vi "TC1016_DEMO.vi"() -> ()   [LabVIEW 2019]
uses:
  SubVI/Typedef/TLibLIN.ctl
panel:
  out "Connect_TSLIN_Successfully":bool
  in  "退出程序":bool
  in  "打开LIN":bool
  in  "选项卡控件":T1(tab)
  in  "TLIBLIN 2":T2
  in  "LIN1_Write":bool
  in  "LIN1_ABaudrateKbps":sgl=19.2 format="%#_g  k"
  in  "LIN1_AProtocol":i32(ring)=2 items=["Lin_Protocol_13", "Lin_Protocol_20", "Lin_Protocol_21", "Lin_Protocol_J2602"]
  in  "LIN1_AHwChannel":i32(ring) items=["CHN1", "CHN2", "CHN3", "CHN4", "CHN5", "CHN6", "CHN7", "CHN8", "CHN9", "CHN10", "CHN11", "CHN12", "CHN13", "CHN14", "CHN15", "CHN16", "CHN17", "CHN18", "CHN19", "CHN20", "CHN21", "CHN22", "CHN23", "CHN24", "CHN25", "CHN26", "CHN27", "CHN28", "CHN29", "CHN30", "CHN31", "CHN32"]
  in  "LIN1_AAppChannel":i32(ring) items=["CHN1", "CHN2", "CHN3", "CHN4", "CHN5", "CHN6", "CHN7", "CHN8", "CHN9", "CHN10", "CHN11", "CHN12", "CHN13", "CHN14", "CHN15", "CHN16", "CHN17", "CHN18", "CHN19", "CHN20", "CHN21", "CHN22", "CHN23", "CHN24", "CHN25", "CHN26", "CHN27", "CHN28", "CHN29", "CHN30", "CHN31", "CHN32"]
  in  "LIN1_SetNode":i32(ring) items=["MasterNode", "SlaveNode", "MonitorNote"]
  in  "启用4通道":bool
  in  "启用3通道":bool
  in  "启用2通道":bool
  in  "启用1通道":bool
  in  "使用通道数量":u16(ring)=1 items=["1通道"=1, "2通道"=2, "3通道"=3, "4通道"=4, "5通道"=5]
  # "TC_1026_DEMO"
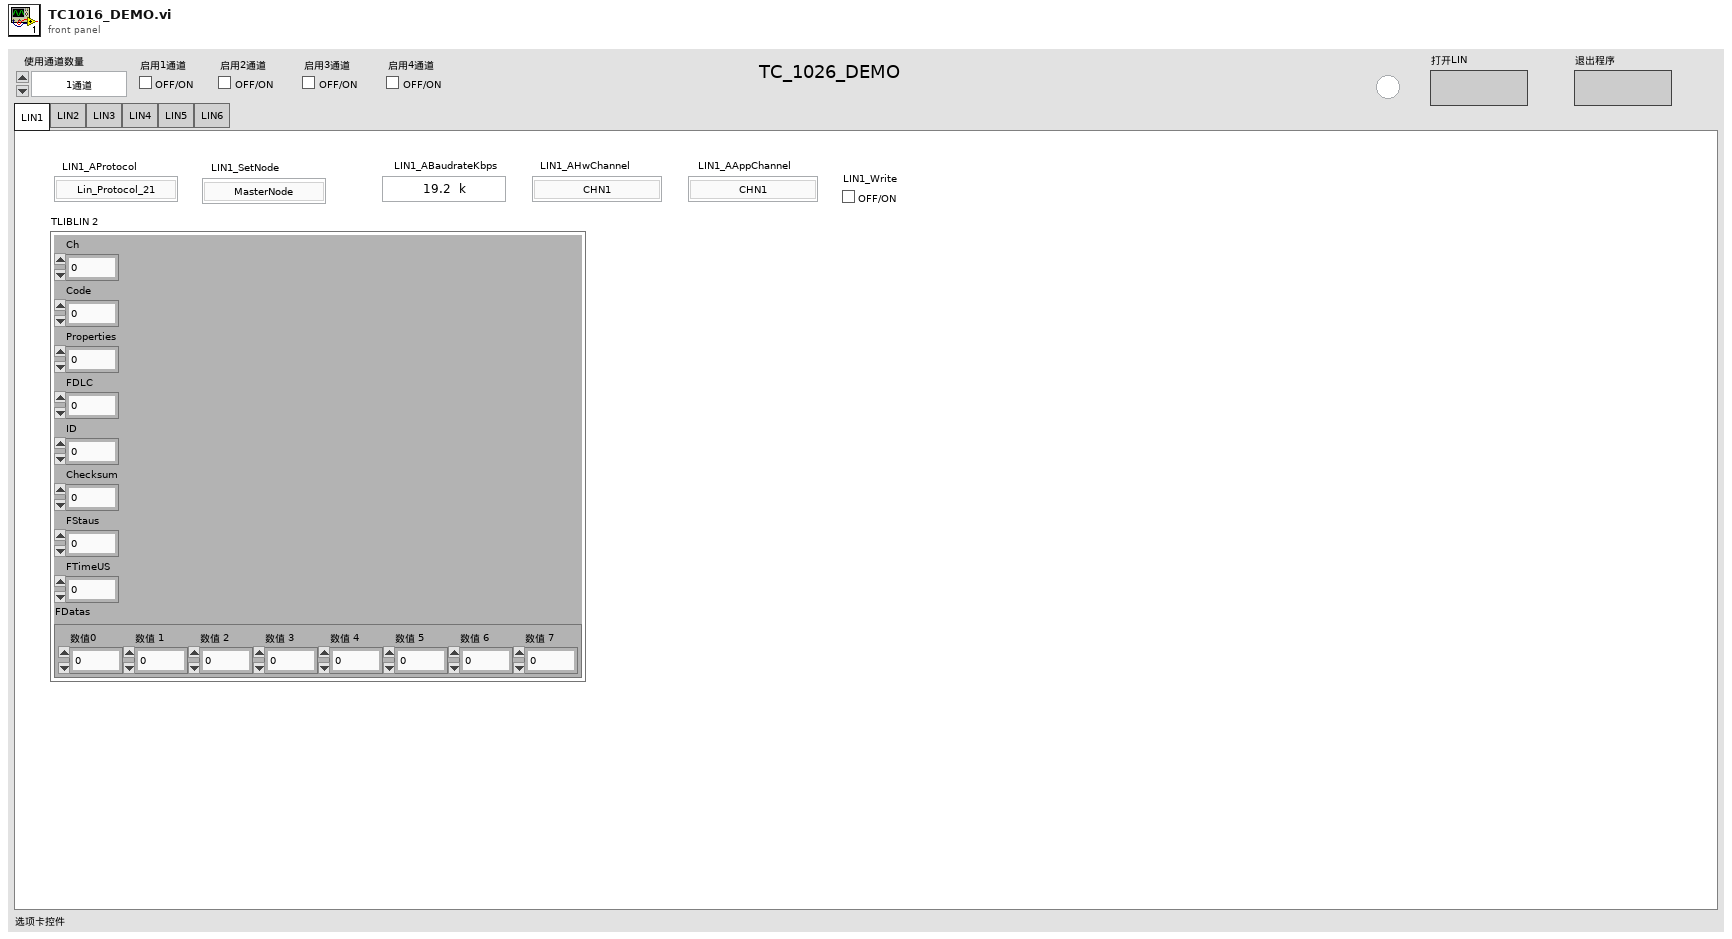
[diagram p1: front panel]
types:
  T1 = enum32{"LIN1", "LIN2", "LIN3", "LIN4", "LIN5", "LIN6"}
  T2 = typedef "TLibLIN.ctl" = cluster{"Ch":u8, "Code":u8, "Properties":u8, "FDLC":u8, "ID":u8, "Checksum":u8, "FStaus":u8, "FTimeUS":u64, "FDatas":cluster{"数值0":u8, "数值 1":u8, "数值 2":u8, "数值 3":u8, "数值 4":u8, "数值 5":u8, "数值 6":u8, "数值 7":u8}}
  T3 = cluster{"硬件类型":i32, "硬件子类型":i32, "AHwChannel":i32, "AAppChannel":i32, "ABaudrateKbps":sgl, "AProtocol":i32}
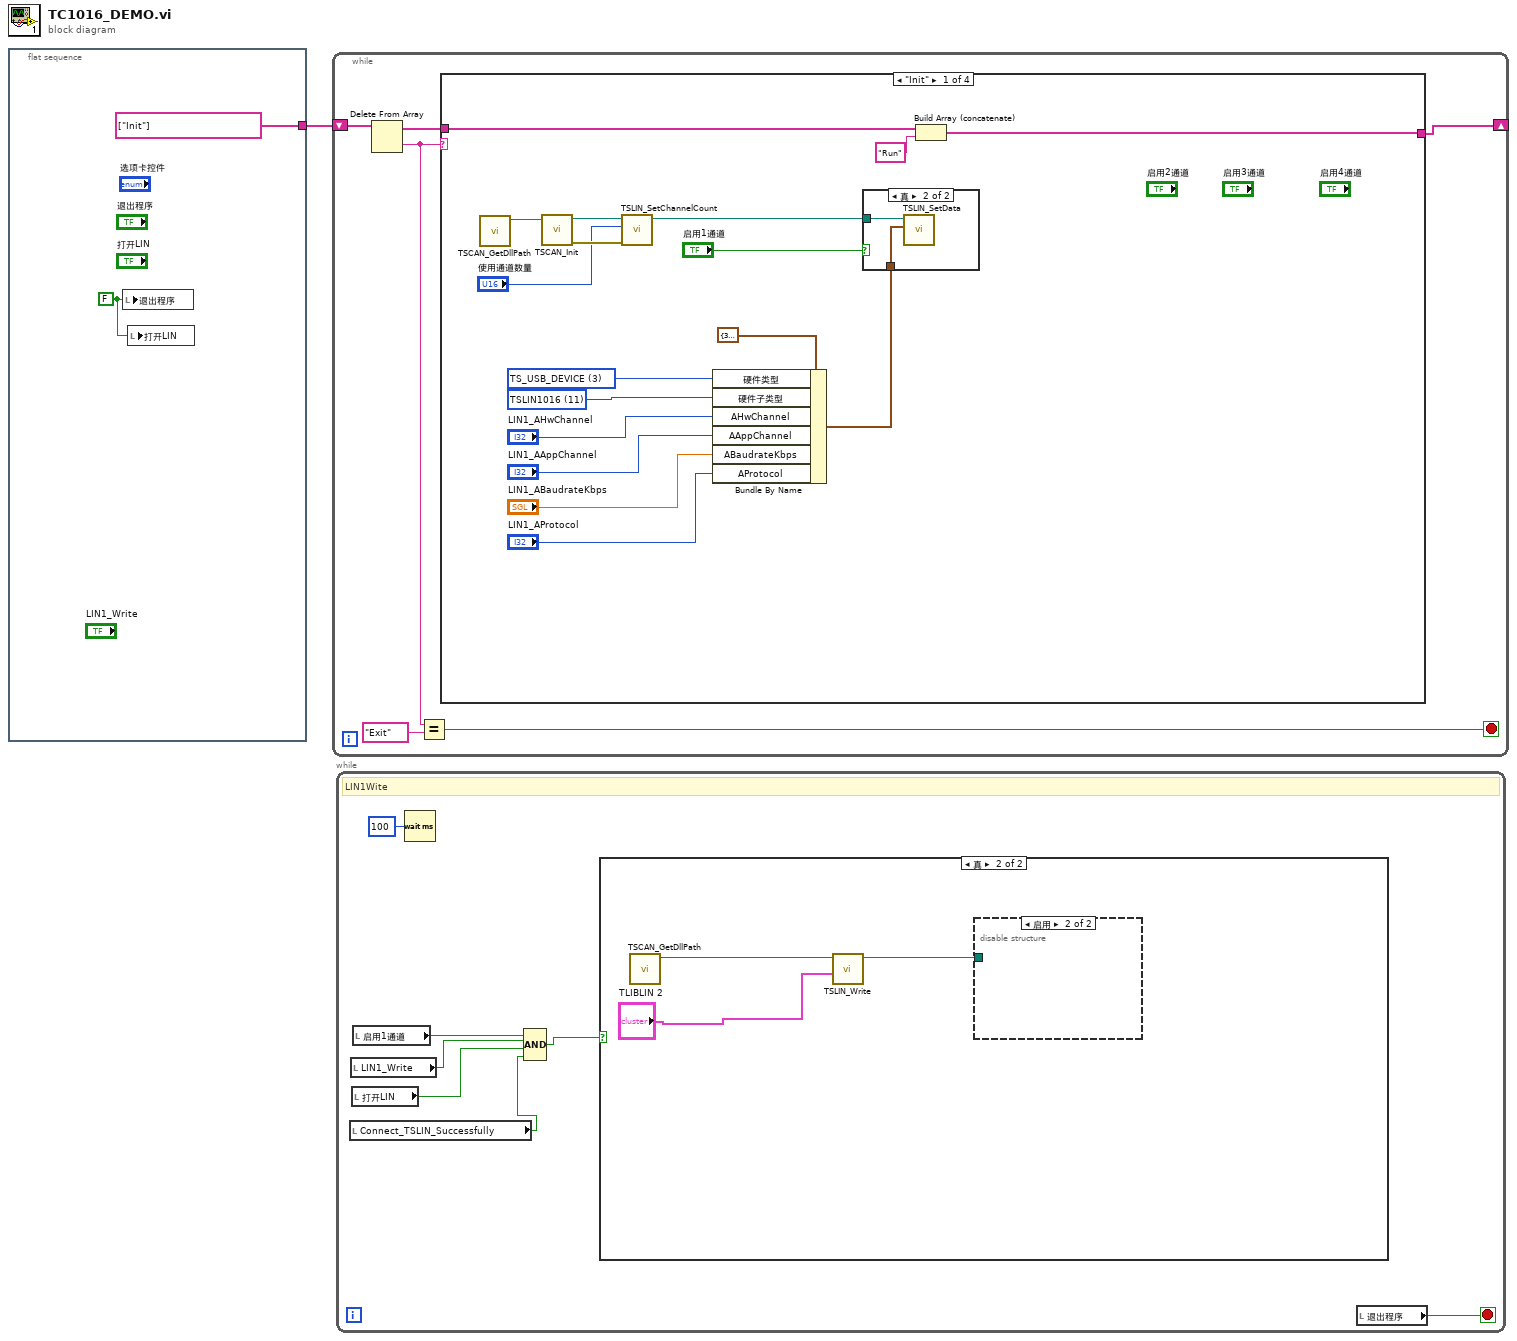
[diagram p0: block diagram]
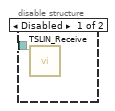
[diagram p3: hidden frame]
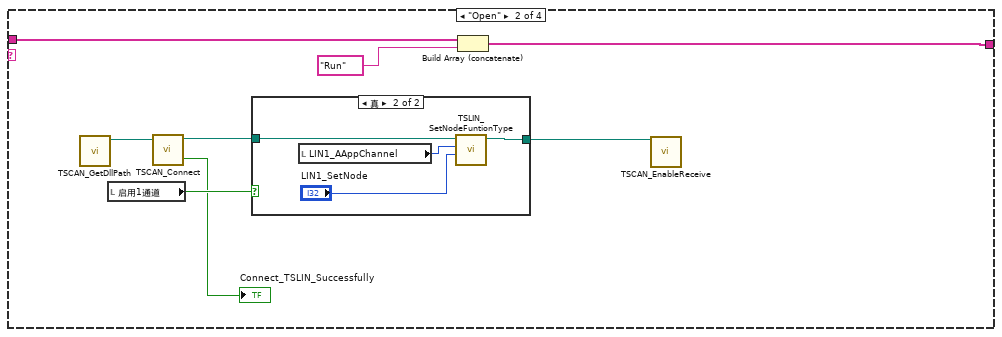
[diagram p5: hidden frame]
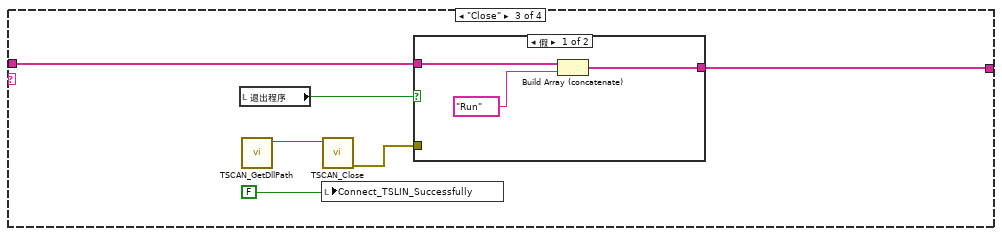
[diagram p7: hidden frame]
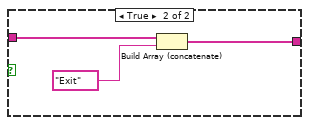
[diagram p8: hidden frame]
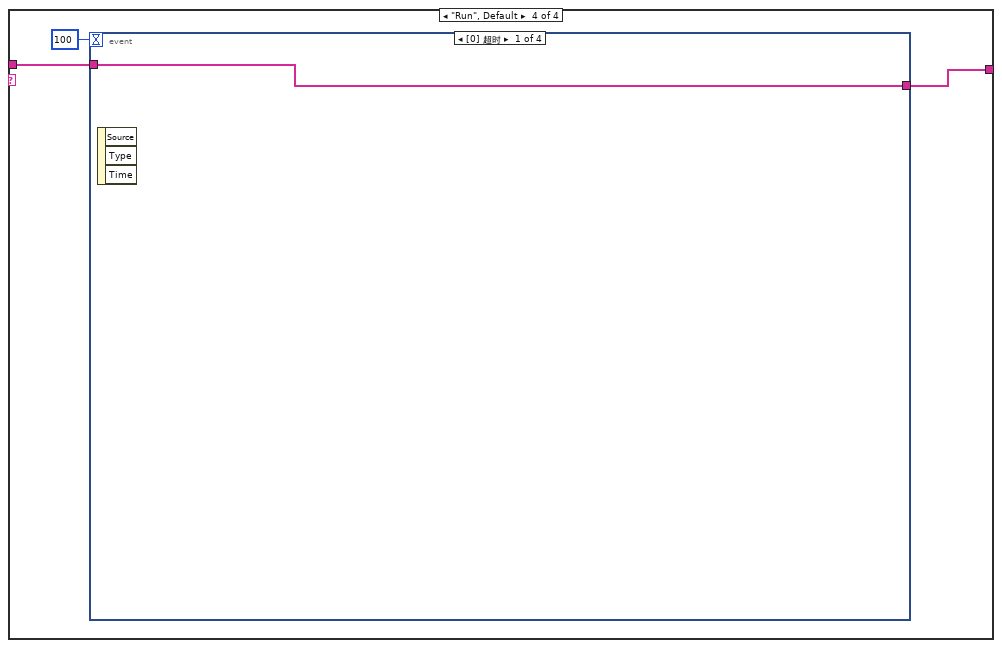
[diagram p9: hidden frame]
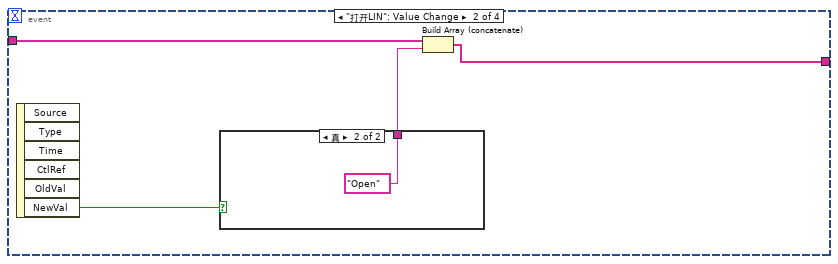
[diagram p10: hidden frame]
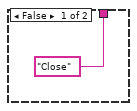
[diagram p11: hidden frame]
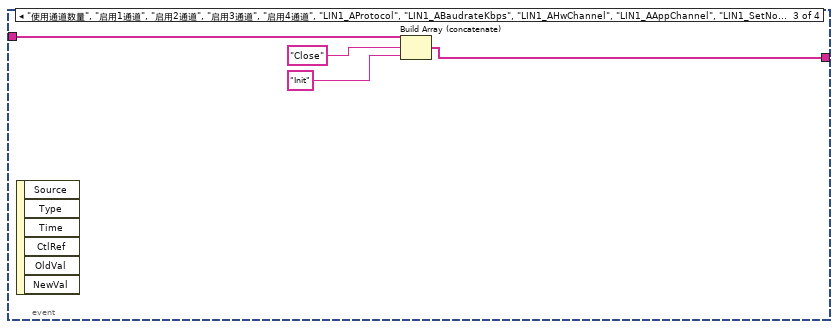
[diagram p12: hidden frame]
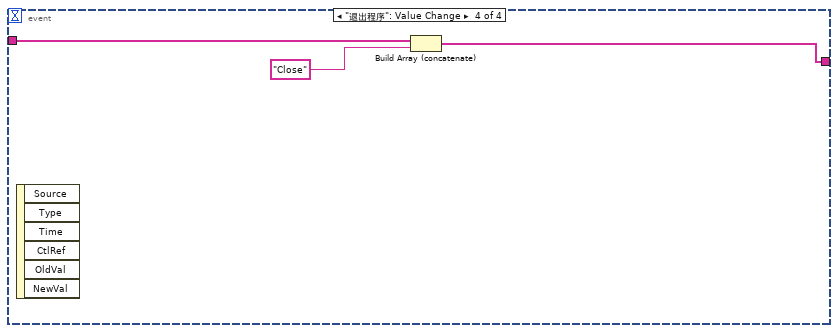
[diagram p13: hidden frame]
diagram:
  n1 = flat-sequence {
    tunnel: [string[] ["Init"]] -> w1
    frame #0 {
      w2 = FALSE ("退出程序")
      n2 = local write "退出程序"(w2) -> ()
      n3 = local write "打开LIN"(w2) -> ()
    }
  }
  n4 = while {
    shift-right: [w8] -> _
    shift-left: w1 -> [w9]
    stop <- w4 stop-if-true
    n5 = Delete From Array(array=w9) -> (deleted portion=w5:string, array with subset deleted=w7:string[])  [unwired: 2 in]
    n6 = Equal?(x=w5, y="Exit") -> (x = y?=w4:bool)
    n7 = case shown="\"Init\"" w5 {
      tunnel: [w25 w34 w43 w54] -> w8
      tunnel: w7 -> [w10 w36 w46 w55]
      frame "Init" {
        w15 = 11 items=["BUS_UNKNOWN_TYPE", "TSCAN_PRO_4", "TSCAN_LITE_2", "TSCANMini", "TSLinMini", "TSCANFDmini", "TSCAN_LIN_IO_2", "TSCAN_LITE_2", "TSCANLIN", "TSCAN_FD_Mini_1", "TSLIN1026", "TSLIN1016"] ("硬件子类型")
        w14 = 3 items=["BUS_UNKNOWN_TYPE", "TS_TCP_DEVICE", "XL_USB_DEVICE", "TS_USB_DEVICE", "PEAK_USB_DEVICE", "KVASER_USB_DEVICE", "ZLG_USB_DEVICE", "ICS_USB_DEVICE", "TS_TC1005_DEVICE"] ("硬件类型")
        n8 = call "TSCAN_GetDllPath.vi"() -> ("DllPath"=w22:path)  [unwired: 11 in]
        n9 = call "TSCAN_Init.vi"("路径输入"=w22) -> ("错误输出"=w24:errorcluster, "路径输出"=w23:path)  [unwired: 8 in, 1 out]
        n10 = call "TSLIN_SetChannelCount.vi"("错误输入（无错误）"=w24, "Aount"="使用通道数量", "路径输入"=w23) -> ("路径输出"=w20:path)  [unwired: 6 in, 2 out]
        n11 = Bundle By Name(cluster=T3 {"硬件类型"=3, "硬件子类型"=10, "AHwChannel"=0, "AAppChannel"=0, "ABaudrateKbps"=19.2, "AProtocol"=2} ("Set"), "硬件类型"=w14, "硬件子类型"=w15, "AHwChannel"="LIN1_AHwChannel", "AAppChannel"="LIN1_AAppChannel", "ABaudrateKbps"="LIN1_ABaudrateKbps", "AProtocol"="LIN1_AProtocol") -> (w11:T3)
        n12 = case shown="真" "启用1通道" {
          tunnel: w20 -> [_ w28]
          tunnel: w11 -> [_ w27]
          frame False {
          }
          frame True {
            n13 = call "TSLIN_SetData.vi"("Set"=w27, "路径输入"=w28) -> ()  [unwired: 6 in, 4 out]
          }
        }
        n14 = Build Array (concatenate)(w10, "Run" ("元素")) -> (w25:string[])
      }
      frame "Open" {
        n15 = call "TSCAN_GetDllPath.vi"() -> ("DllPath"=w33:path)  [unwired: 11 in]
        n16 = local read "启用1通道"() -> (w31:bool)
        n17 = call "TSCAN_Connect.vi"("路径输入"=w33) -> ("路径输出"=w32:path, "Connect_TSCAN_Successfully"=→"Connect_TSLIN_Successfully":bool)  [unwired: 8 in, 1 out]
        n18 = case shown="真" w31 {
          tunnel: w32 -> [w37 w41]
          tunnel: [w37 w40] -> w30
          frame False {
          }
          frame True {
            n19 = local read "LIN1_AAppChannel"() -> (w39:i32)
            n20 = call "TSLIN_SetNodeFuntionType.vi"("set_node_funtiontype"="LIN1_SetNode", "AAppChannel"=w39, "路径输入"=w41) -> ("路径输出"=w40:path)  [unwired: 8 in]
          }
        }
        n21 = Build Array (concatenate)(w36, "Run") -> (w34:string[])
        n22 = call "TSCAN_EnableReceive.vi"("路径输入"=w30) -> ()  [unwired: 9 in, 2 out]
      }
      frame "Close" {
        n23 = local read "退出程序"() -> (w44:bool)
        n24 = call "TSCAN_GetDllPath.vi"() -> ("DllPath"=w47:path)  [unwired: 11 in]
        n25 = local write "Connect_TSLIN_Successfully"(FALSE ("Connect_TSLIN_Successfully")) -> ()
        n26 = call "TSCAN_Close.vi"("路径输入"=w47) -> ("错误输出"=w45:errorcluster)  [unwired: 9 in, 1 out]
        n27 = case shown="假" w44 {
          tunnel: [w48 w52] -> w43
          tunnel: w46 -> [w49 w51]
          tunnel: w45 -> [_ _]
          frame False {
            n28 = Build Array (concatenate)(w49, "Run") -> (w48:string[])
          }
          frame True {
            n29 = Build Array (concatenate)(w51, "Exit") -> (w52:string[])
          }
        }
      }
      frame "Run", Default {
        n30 = event shown="[0] 超时" {
          selector: _ -> [_ _ _ _]
          dyn-events: _ -> [_ _ _ _]
          timeout: 100 -> [_ _ _ _]
          tunnel: w55 -> [w57 w60 w66 w70]
          tunnel: [w57 w59 w67 w69] -> w54
          event Timeout {
            n31 = event-data() -> ()  [unwired: 1 in, 3 out]
          }
          event "打开LIN": Value Change {
            n32 = event-data() -> ("NewVal"=w61:bool)  [unwired: 1 in, 5 out]
            n33 = case shown="真" w61 {
              tunnel: ["Close" "Open"] -> w58
              frame False {
              }
              frame True {
              }
            }
            n34 = Build Array (concatenate)(w60, w58) -> (w59:string[])
          }
          event "使用通道数量", "启用1通道", "启用2通道", "启用3通道", "启用4通道", "LIN1_AProtocol", "LIN1_ABaudrateKbps", "LIN1_AHwChannel", "LIN1_AAppChannel", "LIN1_SetNode": Value Change {
            n35 = event-data() -> ()  [unwired: 1 in, 6 out]
            n36 = Build Array (concatenate)(w66, "Close", "Init") -> (w67:string[])
          }
          event "退出程序": Value Change {
            n37 = event-data() -> ()  [unwired: 1 in, 6 out]
            n38 = Build Array (concatenate)(w70, "Close") -> (w69:string[])
          }
        }
      }
    }
  }
  n39 = while {
    stop <- w77 stop-if-true
    # "LIN1Wite"
    n40 = local read "Connect_TSLIN_Successfully"() -> (w71:bool)
    n41 = local read "LIN1_Write"() -> (w73:bool)
    n42 = local read "打开LIN"() -> (w72:bool)
    n43 = local read "启用1通道"() -> (w74:bool)
    n44 = Wait (ms)(milliseconds to wait=u32 100 ("等待时间（毫秒）")) -> ()  [unwired: 1 out]
    n45 = Compound Arithmetic op=AND ("复合运算")(w74, w73, w72, w71) -> (w75:bool)
    n46 = case shown="真" w75 {
      frame False {
      }
      frame True {
        n47 = call "TSCAN_GetDllPath.vi"() -> ("DllPath"=w80:path)  [unwired: 11 in]
        n48 = call "TSLIN_Write.vi"("TLIBLIN"="TLIBLIN 2", "路径输入"=w80) -> ("路径输出"=w79:path)  [unwired: 7 in, 2 out]
        n49 = disable-structure shown="启用" {
          disable-tunnel: w79 -> [w81 _]
          frame Disabled {
            n50 = call "TSLIN_Receive.vi"("路径输入"=w81) -> ()  [unwired: 9 in, 1 out]
          }
          frame Enabled {
          }
        }
      }
    }
    n51 = local read "退出程序"() -> (w77:bool)
  }
